vi "RandBigInt.vi"(1 "length (x1e9)":i16) -> (0 "Random Number":cluster{"P/N":bool, "Array":u64[]})   [LabVIEW 2023]
uses:
  <vilib>/numeric/Random Number (Range) U64.vi
  <vilib>/numeric/sub_Random U32.vi
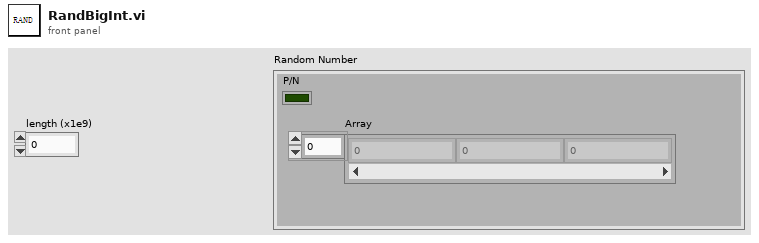
[diagram p1: front panel]
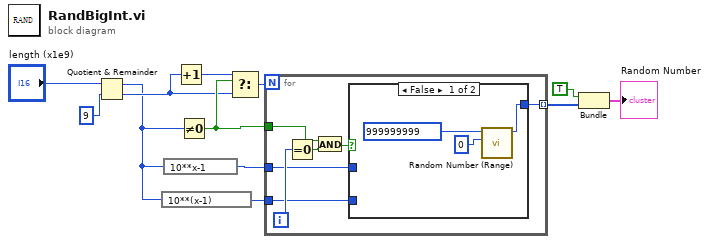
[diagram p0: block diagram]
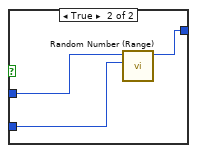
[diagram p2: hidden frame]
diagram:
  n1 = Quotient & Remainder(x="length (x1e9)", y=9) -> (x-y*floor(x/y)=w2:i32, floor(x/y)=w4:i32)
  n2 = expression code="10**(x-1)"(w2) -> (w1:i32)
  n3 = expression code="10**x-1"(w2) -> (w7:i32)
  n4 = Increment(x=w4) -> (x+1=w3:i32)
  n5 = Not Equal To 0?(x=w2) -> (x != 0?=w5:bool)
  n6 = Select(t=w3, s=w5, f=w4) -> (s? t:f=w6:i32)
  n7 = for {
    N: w6 -> [_]
    tunnel: [w19] -> w11 mode=indexing
    tunnel: w7 -> [w17]
    tunnel: w5 -> [w16]
    tunnel: w1 -> [w13]
    i -> [w18]
    n8 = Equal To 0?(x=w18) -> (x = 0?=w15:bool)
    n9 = And(x=w16, y=w15) -> (x .and. y?=w14:bool)
    n10 = case shown="False" w14 {
      tunnel: [w20 w24] -> w19
      tunnel: w17 -> [_ w25]
      tunnel: w13 -> [_ w23]
      frame False {
        n11 = call-poly <vilib>:"Random Number (Range).vi"("lower bound (0)"=0, "upper bound (100)"=u32 999999999) -> ("number"=w20:u64)  [unwired: 9 in]
      }
      frame True {
        n12 = call-poly <vilib>:"Random Number (Range).vi"("lower bound (0)"=w23, "upper bound (100)"=w25) -> ("number"=w24:u64)  [unwired: 9 in]
      }
    }
  }
  n13 = Bundle(TRUE, w11) -> (→"Random Number":cluster{bool, u64[]})  [unwired: 1 in]
